vi "4155C Take SampleI.vi"(7 "Emergency Stop":refnum<vi>, 8 "error in (no error)":errorcluster, 9 "Idg 2":dbl min=-100.0 max=100.0 format="%.15e", 10 "Vdg compliance 2":dbl min=-100.0 max=100.0 format="%.15e", 11 "VISA resource name in":refnum<visa-resource-name>) -> (0 "error out":errorcluster, 1 "Idg":dbl[](array[numeric]) format="%.2f", 2 "Vdg":dbl[](array[numeric]) format="%.2f", 3 "VISA Resource Name out":refnum<visa-resource-name>, 4 "Is":dbl[](array[numeric]) format="%.2f", 5 "Time":dbl[](array[numeric]) format="%.2f")   [LabVIEW 2016]
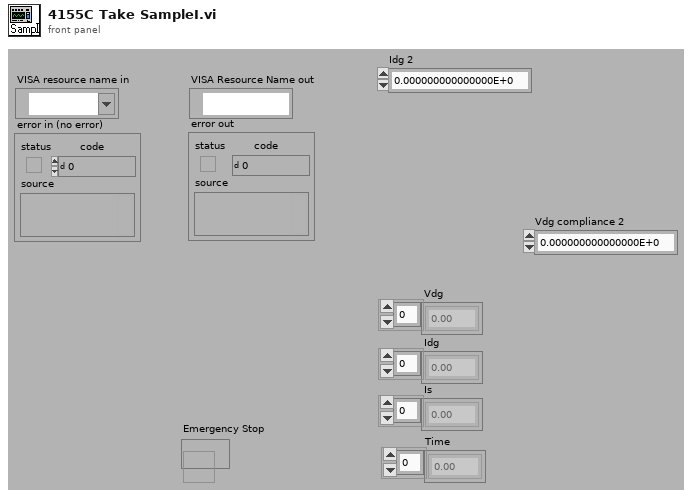
[diagram p1: front panel]
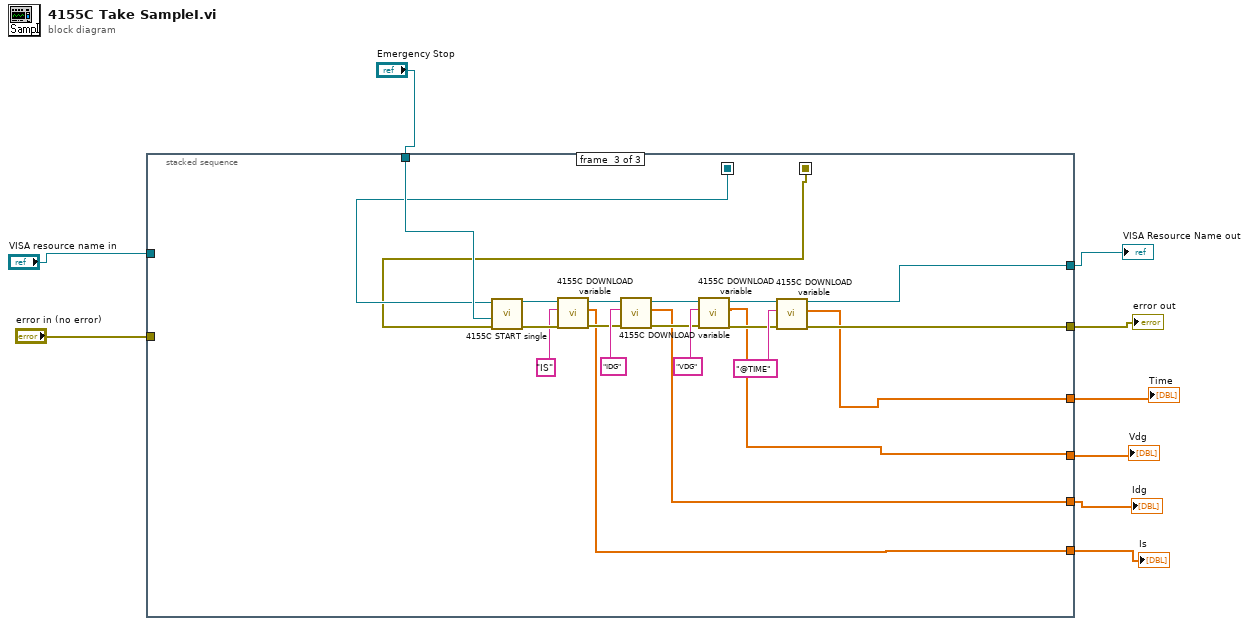
[diagram p0: block diagram]
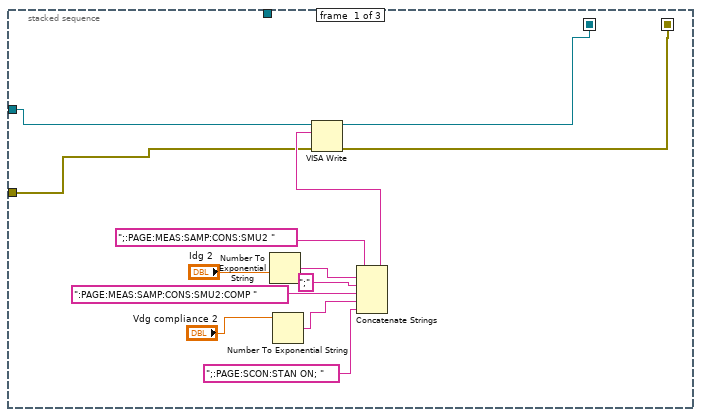
[diagram p2: hidden frame]
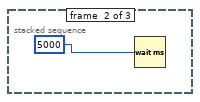
[diagram p3: hidden frame]
diagram:
  n1 = stacked-sequence {
    seq-local: [w11 _ _] -> [_ _ w25]
    seq-local: [w10 _ _] -> [_ _ w24]
    tunnel: "Emergency Stop" -> [_ _ w32]
    tunnel: "VISA resource name in" -> [w14 _ _]
    tunnel: "error in (no error)" -> [w13 _ _]
    tunnel: [_ _ w31] -> w6
    tunnel: [_ _ w30] -> w5
    tunnel: [_ _ w29] -> w4
    tunnel: [_ _ w28] -> w3
    tunnel: [_ _ w27] -> w2
    tunnel: [_ _ w26] -> w1
    frame #0 {
      n2 = Number To Exponential String(number="Idg 2") -> (E-format string=w16:string)  [unwired: 3 in]
      n3 = Number To Exponential String(number="Vdg compliance 2") -> (E-format string=w20:string)  [unwired: 3 in]
      n4 = Concatenate Strings(";:PAGE:MEAS:SAMP:CONS:SMU2 " ("write buffer (\"\")"), w16, ";" ("Substring"), ":PAGE:MEAS:SAMP:CONS:SMU2:COMP " ("write buffer (\"\")"), w20, ";:PAGE:SCON:STAN ON; " ("write buffer (\"\")")) -> (w17:string)
      n5 = VISA Write(VISA resource name=w14, write buffer=w17, error in (no error)=w13) -> (VISA resource name out=w11:refnum<visa-resource-name>, error out=w10:errorcluster)  [unwired: 1 out]
    }
    frame #1 {
      n6 = Wait (ms)(milliseconds to wait=5000) -> ()  [unwired: 1 out]
    }
    frame #2 {
      n7 = call "4155C START single.vi"("error in (no error)"=w24, "Emergency Stop"=w32, "VISA resource name in"=w25) -> ("error out"=w43:errorcluster, "VISA Resource Name out"=w44:refnum<visa-resource-name>)  [unwired: 3 in]
      n8 = call "4155C DOWNLOAD variable.vi"("error in (no error)"=w43, "Variable name"="IS", "VISA resource name in"=w44) -> ("error out"=w40:errorcluster, "Output data"=w26:dbl[], "VISA Resource Name out"=w39:refnum<visa-resource-name>)  [unwired: 2 in]
      n9 = call "4155C DOWNLOAD variable.vi"("error in (no error)"=w40, "Variable name"="IDG", "VISA resource name in"=w39) -> ("error out"=w37:errorcluster, "Output data"=w27:dbl[], "VISA Resource Name out"=w36:refnum<visa-resource-name>)  [unwired: 2 in]
      n10 = call "4155C DOWNLOAD variable.vi"("error in (no error)"=w37, "Variable name"="VDG", "VISA resource name in"=w36) -> ("error out"=w33:errorcluster, "Output data"=w28:dbl[], "VISA Resource Name out"=w34:refnum<visa-resource-name>)  [unwired: 2 in]
      n11 = call "4155C DOWNLOAD variable.vi"("error in (no error)"=w33, "Variable name"="@TIME", "VISA resource name in"=w34) -> ("error out"=w30:errorcluster, "Output data"=w29:dbl[], "VISA Resource Name out"=w31:refnum<visa-resource-name>)  [unwired: 2 in]
    }
  }
  "VISA Resource Name out" <- w6
  "error out" <- w5
  "Time" <- w4
  "Vdg" <- w3
  "Idg" <- w2
  "Is" <- w1
